vi "Test Report Contain TestCase Time.vi"(8 "error in (no error)":errorcluster, 11 "XML Report Test in":refnum<class "XML Report Test.lvclass">) -> (0 "error out":errorcluster, 3 "XML Report Test out":refnum<class "XML Report Test.lvclass">)   [LabVIEW 2020, in "XML Report Test.lvclass"]
uses:
  XML Report Test.lvclass
  XML Report Test.lvclass/XML Report Test.ctl
  source/Plugins/XML Report/XML Report.lvclass
panel:
  out "Report Content":string
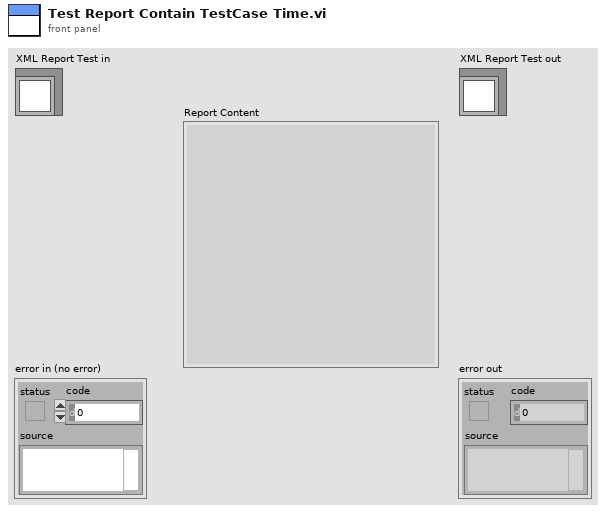
[diagram p1: front panel]
types:
  T1 = typedef "Result.lvlib/Result.ctl" = cluster{"Name":string, "Message":string, "Description":string, "Status":T2, "Result Type":T3, "Execution Time":dbl}
  T2 = typedef "Result.lvlib/Status.ctl" = enum16{"", "Passed", "Failed", "Error", "Skipped", "Setup Error", "Broken", "Teardown Error"}
  T3 = typedef "Result.lvlib/Type.ctl" = enum16{"Method", "Case", "Suite", "Pass", "Fail", "Skip", "Pass if", "Fail if", "Pass if Error", "Fail if Error", "Pass if Equal", "Fail if Equal"}
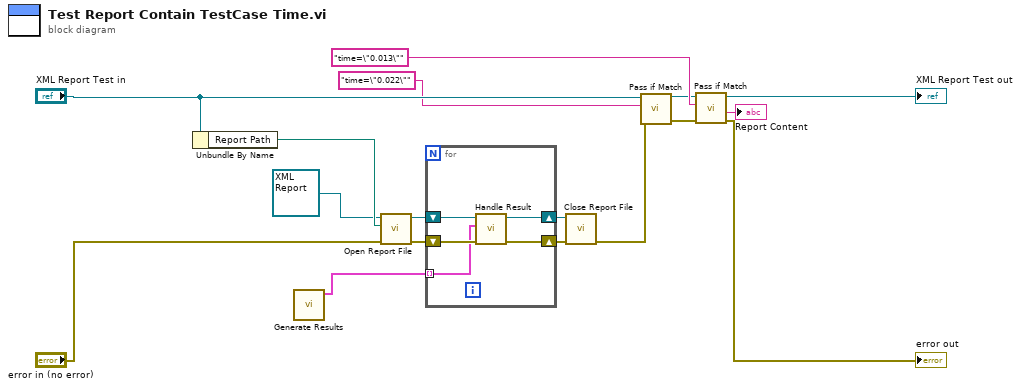
[diagram p0: block diagram]
diagram:
  n1 = Unbundle By Name("XML Report Test in") -> ("Report Path"=w12:path)
  n2 = call "Generate Results.vi"() -> ("Data"=w6:T1[])  [unwired: 10 in, 1 out]
  n3 = call-dynamic "Open Report File.vi"("error in (no error)"="error in (no error)", "Report Path"=w12, "XML Report In"=refnum<class "XML Report.lvclass"> refnum) -> ("error out"=w17:errorcluster, "XML Report Out"=w8:refnum<class "XML Report.lvclass">)  [unwired: 7 in]
  n4 = for {
    shift-right: [w21] -> w9
    shift-left: w17 -> [w22]
    shift-right: [w19] -> w7
    shift-left: w8 -> [w20]
    tunnel: w6 -> [w18] mode=indexing
    n5 = call-dynamic "Handle Result.vi"("error in (no error)"=w22, "Result"=w18, "XML Report In"=w20) -> ("error out"=w21:errorcluster, "XML Report Out"=w19:refnum<class "XML Report.lvclass">)  [unwired: 7 in]
  }
  n6 = call-dynamic "Close Report File.vi"("error in (no error)"=w9, "XML Report In"=w7) -> ("error out"=w14:errorcluster)  [unwired: 9 in]
  n7 = call "Pass if Match.vi"("error in (no error)"=w14, "regular expression"="time=\"0.022\"", "XML Report Test in"="XML Report Test in") -> ("error out"=w4:errorcluster, "XML Report Test out"=w3:refnum<class "XML Report Test.lvclass">)  [unwired: 6 in, 1 out]
  n8 = call "Pass if Match.vi"("error in (no error)"=w4, "regular expression"="time=\"0.013\"", "XML Report Test in"=w3) -> ("error out"=→"error out":errorcluster, "Report Content"=→"Report Content":string, "XML Report Test out"=→"XML Report Test out":refnum<class "XML Report Test.lvclass">)  [unwired: 6 in]
